vi "Ic distribution simulation.vi"() -> ()   [LabVIEW 2023]
uses:
  paramaters2.ctl
panel:
  in  "Tab Control":T1(tab)
  out "Escaping rate plots":cluster{"I":dbl[], "MQT":dbl[]}[](graph)
  out "Ic T+M SD":dbl
  out "Ic TA+MQT data":dbl[](array[numeric])
  out "Ic MQT SD":dbl format="%#.4e"
  out "Ic MQT mean":dbl format="%#.4e"
  out "Ic MQT data":dbl[](array[numeric])
  out "Ic TA SD":dbl format="%#_4e"
  out "Ic TA mean":dbl format="%#.4e"
  out "Ic TA data":dbl[](array[numeric])
  out "Progress":string
  in  "dist run":bool
  out "Ic distribution":T2(graph)
  in  "intervals":i32=47
  out "Ic T+M mean":dbl format="%#.4e"
  out "Ic TA Skewness":dbl format="%#_4e"
  out "Ic MQT Skewness":dbl format="%#_4e"
  out "Ic T+M Skewness":dbl format="%#_4e"
  out "error out":errorcluster
  in  "Stop":bool
  in  "Parameters":T3={"temperature K"=0.05, "C0 capacitance F"=5e-13, "Ic A"=4e-06, "R Ohm"=18.0, "Parity Mode"=enum."Parity with random lifetime", "Parity switch fre"=10000.0, "Parity ratio"=0.5, "Imax A"=5e-06, "Tsw s"=0.01, "N_steps"=10000, "Ic_d"=0.02, "N_sweeps"=10000, "Ic_cut"=0.9} {"temperature K" step=0.01}
  # "v1.91"
  # "Change the values will cause\nupdate of escaping plots."
  # "Instruction:\n\nParity_ratio means the time over total the system in Ic-d/2 state, system will be in random state according to the Parity_ratio before start simulation of each event.\nAssume the current ramp start from zero to Imax for Tsw of time (Ic should be smaller or equal to Imax). The whole ramp contains N_steps. The distribution contains N_sweeps, and assume escaping rate is zero below Ic_cut*Ic"
  # "Use the \"cross\" to close, stop button for developing only."
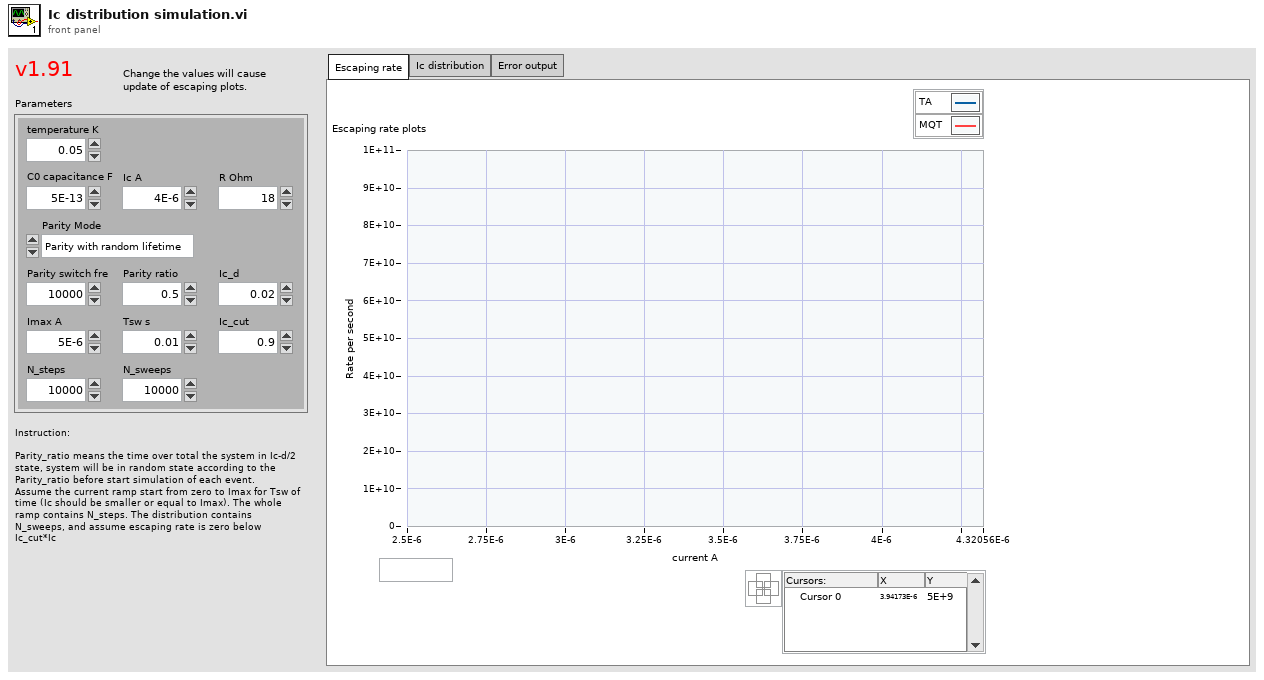
[diagram p1: front panel]
types:
  T1 = enum32{"Escaping rate", "Ic distribution", "Error output"}
  T2 = cluster{"X Values":dbl[], "Histogram: h(x)":i32[]}[]
  T3 = typedef "paramaters2.ctl" = cluster{"temperature K":dbl, "C0 capacitance F":dbl, "Ic A":dbl, "R Ohm":dbl, "Parity Mode":enum16{"No parity", "Parity with random lifetime", "For Ic-Ic_d/2", "For Ic+Ic_d/2", "Parity with constant lifetime"}, "Parity switch fre":dbl, "Parity ratio":dbl, "Imax A":dbl, "Tsw s":dbl, "N_steps":i32, "Ic_d":dbl, "N_sweeps":i32, "Ic_cut":dbl}
  T4 = enum8{"Enabled", "Disabled", "Disabled and Grayed Out"}
  T5 = cluster{"X Values":dbl[], "Histogram: h(x)":i32[]}
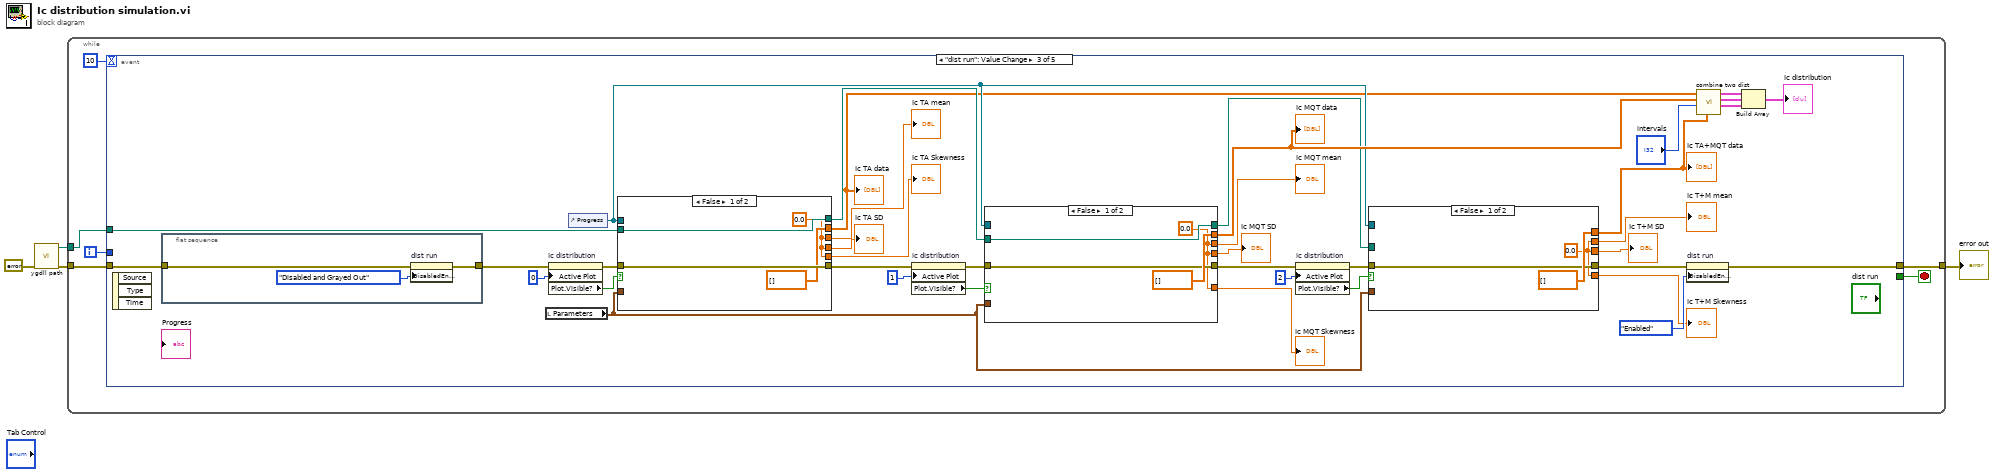
[diagram p0: block diagram]
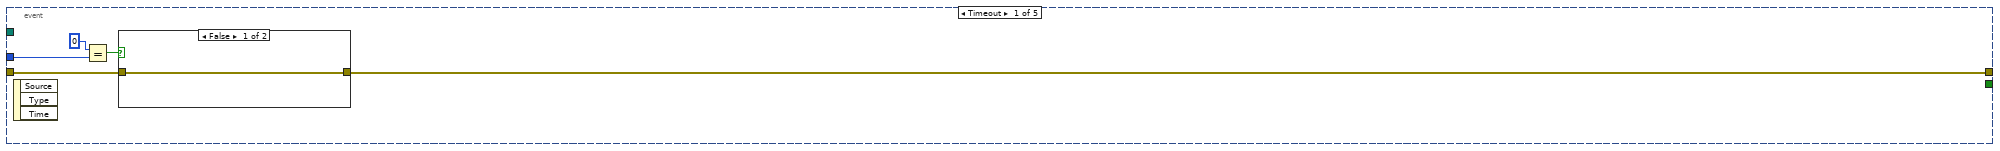
[diagram p2: hidden frame]
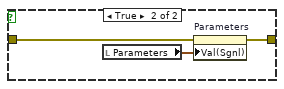
[diagram p3: hidden frame]
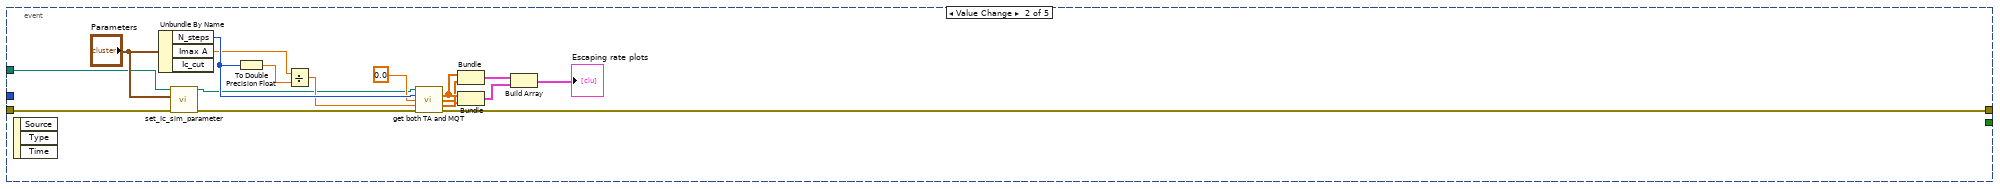
[diagram p4: hidden frame]
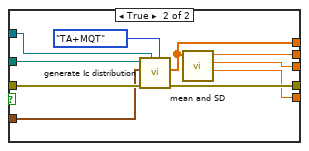
[diagram p5: hidden frame]
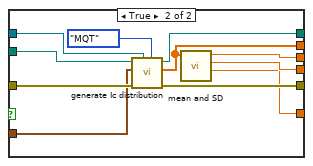
[diagram p6: hidden frame]
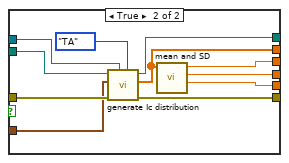
[diagram p7: hidden frame]
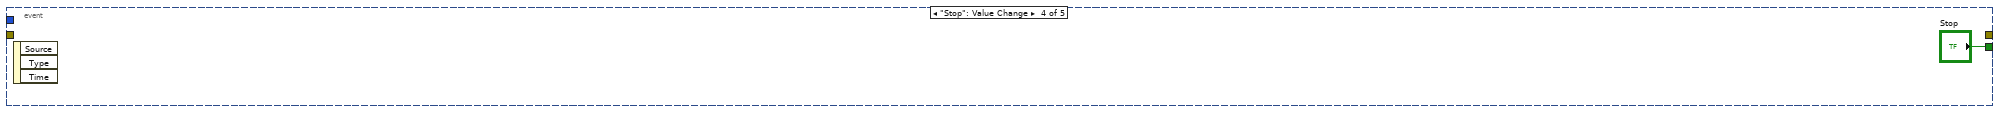
[diagram p8: hidden frame]
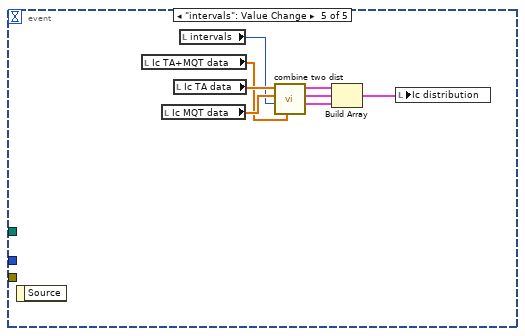
[diagram p9: hidden frame]
diagram:
  n1 = call "ygdll path.vi"("error in (no error)"=errorcluster {"status"=FALSE, "code"=0, "source"=""}) -> ("error out"=w1:errorcluster, "appended path"=w2:path)  [unwired: 9 in]
  n2 = while {
    tunnel: w1 -> [w10]
    tunnel: [w9] -> w4
    tunnel: w2 -> [w7]
    i -> [w6]
    stop <- w5 stop-if-true
    n3 = event shown="[2] \"dist run\": Value Change" {
      selector: _ -> [_ _ _ _ _]
      dyn-events: _ -> [_ _ _ _ _]
      timeout: 10 -> [_ _ _ _ _]
      tunnel: w10 -> [w12 w36 w68 _ _]
      tunnel: [w11 w27 w67 _ _] -> w9
      tunnel: w7 -> [_ w22 w74 _ _]
      tunnel: w6 -> [w15 _ _ _ _]
      tunnel: [_ _ _ "Stop" _] -> w5
      event Timeout {
        n4 = event-data() -> ()  [unwired: 1 in, 3 out]
        n5 = Equal?(x=0, y=w15) -> (x = y?=w13:bool)
        n6 = case shown="False" w13 {
          tunnel: w12 -> [w16 w19]
          tunnel: [w16 w18] -> w11
          frame False {
          }
          frame True {
            n7 = local read "Parameters"() -> (w17:T3)
            n8 = property on="Parameters" class="Clust (strict)"(error in=w19, "Val(Sgnl)"=w17) -> (error out=w18:errorcluster)  [unwired: 1 in, 1 out]
          }
        }
      }
      event Value Change {
        n9 = event-data() -> ()  [unwired: 1 in, 3 out]
        n10 = Unbundle By Name("Parameters") -> ("N_steps"=w34:i32, "Imax A"=w25:dbl)  [unwired: 1 out]
        n11 = call "set_Ic_sim_parameter.vi"("error in (no error)"=w36, "Parameters"="Parameters", "path in"=w22) -> ("error out"=w35:errorcluster, "path out"=w21:path)  [unwired: 7 in]
        n12 = To Double Precision Float(number=w34) -> (double precision float=w33:dbl)
        n13 = Divide(x=w25, y=w33) -> (x/y=w32:dbl)
        n14 = call "get both TA and MQT.vi"("path in"=w21, "Points"=w34, "Start current"=0.0, "Step"=w32, "error in (no error)"=w35) -> ("I"=w31:dbl[], "TA"=w30:dbl[], "MQT"=w26:dbl[], "error out"=w27:errorcluster)  [unwired: 6 in, 1 out]
        n15 = Bundle("I"=w31, "TA"=w30) -> (w29:cluster{"I":dbl[], "TA":dbl[]})  [unwired: 1 in]
        n16 = Bundle("I"=w31, "MQT"=w26) -> (w28:cluster{"I":dbl[], "MQT":dbl[]})  [unwired: 1 in]
        n17 = Build Array(w29, w28) -> (→"Escaping rate plots":cluster{"I":dbl[], "MQT":dbl[]}[])
      }
      event "dist run": Value Change {
        n18 = event-data() -> ()  [unwired: 1 in, 3 out]
        n19 = flat-sequence {
          tunnel: w68 -> [w120]
          tunnel: [w119] -> w51
          frame #0 {
            n20 = property on="dist run" class="Bool"(error in=w120, "DisabledEnum"=T4."Disabled and Grayed Out" ("Disabled")) -> (error out=w119:errorcluster)  [unwired: 1 in, 1 out]
          }
        }
        n21 = local read "Parameters"() -> (w57:T3)
        n22 = property on="Ic distribution" class="XYGraph (strict)"(error in=w51, "Active Plot"=u32 0) -> (error out=w50:errorcluster, "Plot.Visible?"=w48:bool)  [unwired: 1 in, 1 out]
        n23 = control-ref of="Progress"() -> (w58:refnum<vi>)
        n24 = case shown="False" w48 {
          tunnel: w74 -> [w106 w117]
          tunnel: [w105 w115] -> w47
          tunnel: [w106 w114] -> w73
          tunnel: w50 -> [w105 w113]
          tunnel: [dbl[] [] ("return type") w108] -> w52
          tunnel: [w103 w112] -> w65
          tunnel: [w103 w111] -> w61
          tunnel: w58 -> [_ w110]
          tunnel: w57 -> [_ w109]
          tunnel: [w103 w107] -> w39
          frame False {
            w103 = 0.0 ("mean")
          }
          frame True {
            n25 = call "generate Ic distribution.vi"("gmode"=enum16{"TA", "MQT", "TA+MQT"}."TA", "progress indicator"=w110, "error in (no error)"=w113, "Parameters"=w109, "path in"=w117) -> ("error out"=w115:errorcluster, "return type"=w108:dbl[], "path out"=w114:path)  [unwired: 4 in]
            n26 = call "mean and SD.vi"("Input"=w108) -> ("skewness"=w107:dbl, "SD"=w112:dbl, "mean"=w111:dbl)  [unwired: 8 in]
          }
        }
        "Ic TA SD" <- w65
        "Ic TA mean" <- w61
        "Ic TA data" <- w52
        "Ic TA Skewness" <- w39
        n27 = property on="Ic distribution" class="XYGraph (strict)"(error in=w47, "Active Plot"=u32 1) -> (error out=w46:errorcluster, "Plot.Visible?"=w44:bool)  [unwired: 1 in, 1 out]
        n28 = case shown="False" w44 {
          tunnel: w46 -> [w89 w102]
          tunnel: w73 -> [w90 w101]
          tunnel: [dbl[] [] ("return type") w99] -> w64
          tunnel: [w88 w98] -> w63
          tunnel: [w88 w97] -> w62
          tunnel: [w89 w96] -> w43
          tunnel: [w90 w95] -> w59
          tunnel: w58 -> [_ w94]
          tunnel: w57 -> [_ w93]
          tunnel: [w88 w92] -> w38
          frame False {
            w88 = 0.0 ("SD")
          }
          frame True {
            n29 = call "generate Ic distribution.vi"("gmode"=enum16{"TA", "MQT", "TA+MQT"}."MQT", "progress indicator"=w94, "error in (no error)"=w102, "Parameters"=w93, "path in"=w101) -> ("error out"=w96:errorcluster, "return type"=w99:dbl[], "path out"=w95:path)  [unwired: 4 in]
            n30 = call "mean and SD.vi"("Input"=w99) -> ("skewness"=w92:dbl, "SD"=w97:dbl, "mean"=w98:dbl)  [unwired: 8 in]
          }
        }
        "Ic MQT data" <- w64
        "Ic MQT mean" <- w63
        "Ic MQT SD" <- w62
        "Ic MQT Skewness" <- w38
        n31 = property on="Ic distribution" class="XYGraph (strict)"(error in=w43, "Active Plot"=u32 2) -> (error out=w42:errorcluster, "Plot.Visible?"=w40:bool)  [unwired: 1 in, 1 out]
        n32 = case shown="False" w40 {
          tunnel: w42 -> [w76 w87]
          tunnel: [w76 w86] -> w60
          tunnel: w59 -> [_ w85]
          tunnel: w58 -> [_ w84]
          tunnel: w57 -> [_ w83]
          tunnel: [dbl[] [] ("return type") w81] -> w55
          tunnel: [w75 w80] -> w54
          tunnel: [w75 w79] -> w53
          tunnel: [w75 w78] -> w37
          frame False {
            w75 = 0.0 ("mean")
          }
          frame True {
            n33 = call "generate Ic distribution.vi"("gmode"=enum16{"TA", "MQT", "TA+MQT"}."TA+MQT", "progress indicator"=w84, "error in (no error)"=w87, "Parameters"=w83, "path in"=w85) -> ("error out"=w86:errorcluster, "return type"=w81:dbl[])  [unwired: 4 in, 1 out]
            n34 = call "mean and SD.vi"("Input"=w81) -> ("skewness"=w78:dbl, "SD"=w79:dbl, "mean"=w80:dbl)  [unwired: 8 in]
          }
        }
        "Ic TA+MQT data" <- w55
        "Ic T+M mean" <- w54
        "Ic T+M SD" <- w53
        "Ic T+M Skewness" <- w37
        n35 = property on="dist run" class="Bool"(error in=w60, "DisabledEnum"=T4."Enabled" ("Disabled")) -> (error out=w67:errorcluster)  [unwired: 1 in, 1 out]
        n36 = call "combine two dist.vi"("Array3"=w55, "# bins"="intervals", "Array2"=w64, "Array1"=w52) -> ("Histogram 3"=w56:T5, "Histogram 2"=w70:T5, "Histogram 1"=w71:T5)  [unwired: 5 in]
        n37 = Build Array(w71, w70, w56) -> (→"Ic distribution":T2)
      }
      event "Stop": Value Change {
        n38 = event-data() -> ()  [unwired: 1 in, 3 out]
      }
      event "intervals": Value Change {
        n39 = event-data() -> ()  [unwired: 1 in, 1 out]
        n40 = local read "Ic TA+MQT data"() -> (w123:dbl[])
        n41 = local read "Ic MQT data"() -> (w127:dbl[])
        n42 = local read "Ic TA data"() -> (w128:dbl[])
        n43 = local read "intervals"() -> (w126:i32)
        n44 = call "combine two dist.vi"("Array3"=w123, "# bins"=w126, "Array2"=w127, "Array1"=w128) -> ("Histogram 3"=w122:T5, "Histogram 2"=w124:T5, "Histogram 1"=w125:T5)  [unwired: 5 in]
        n45 = Build Array(w125, w124, w122) -> (w129:T2)
        n46 = local write "Ic distribution"(w129) -> ()
      }
    }
  }
  "error out" <- w4
